vi "_TangoReadULong64ScalarAttribute.vi"(3 "error in":errorcluster, 4 "attribute name":string, 5 "device name":string) -> (0 "error out":errorcluster, 1 "setpoint":u64, 2 "value":u64)   [LabVIEW 2014, in "tango.lvlib"]
uses:
  tango.lvlib
  Common VIs/Typedefs/_AttributeDataType_t.ctl
  Extractors/base/toULong64Scalar.vi
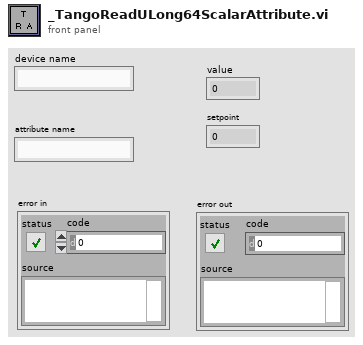
[diagram p1: front panel]
types:
  T1 = typedef "tango.lvlib/_AttributeDataType_t.ctl" = enum16{"STATE_SCA", "STATE_SPE", "STATE_IMG", "STRING_SCA", "STRING_SPE", "STRING_IMG", "BOOL_SCA", "BOOL_SPE", "BOOL_IMG", "UCHAR_SCA", "UCHAR_SPE", "UCHAR_IMG", "SHORT_SCA", "SHORT_SPE", "SHORT_IMG", "USHORT_SCA", "USHORT_SPE", "USHORT_IMG", "LONG_SCA", "LONG_SPE", "LONG_IMG", "ULONG_SCA", "ULONG_SPE", "ULONG_IMG", "LONG64_SCA", "LONG64_SPE", "LONG64_IMG", "ULONG64_SCA", "ULONG64_SPE", "ULONG64_IMG", "FLOAT_SCA", "FLOAT_SPE", "FLOAT_IMG", "DOUBLE_SCA", "DOUBLE_SPE", "DOUBLE_IMG", "ENUM_SCA", "UNKNOWN_DATA_TYPE"}
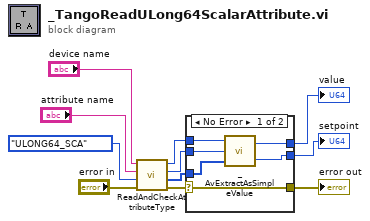
[diagram p0: block diagram]
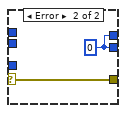
[diagram p2: hidden frame]
diagram:
  n1 = call "ReadAndCheckAttributeType.vi"("error in (no error)"="error in", "expected data type"=_AttributeDataType_t."ULONG64_SCA" ("Control"), "attribute name"="attribute name", "device name"="device name") -> ("error out"=w5:errorcluster, "value"=w9:u8[], "dim. y"=w10:i32, "dim. x"=w11:i32)  [unwired: 4 in]
  n2 = case shown="No Error" w5 {
    selector: w5 -> [w12 w18]
    tunnel: w11 -> [w17 _]
    tunnel: w10 -> [w16 _]
    tunnel: w9 -> [w15 _]
    tunnel: [w14 w19] -> w7
    tunnel: [w13 w19] -> w6
    tunnel: [w12 w18] -> w4
    frame No Error {
      n3 = call-poly "_AvExtractAsSimpleValue.vi"("value_in"=w15, "dim_y"=w16, "dim_x"=w17) -> ("setpoint"=w13:u64, "value"=w14:u64)
    }
    frame Error {
      w19 = u64 0 ("value_out")
    }
  }
  "error out" <- w4
  "value" <- w7
  "setpoint" <- w6
